vi "Test Enr file.vi"() -> ()   [LabVIEW 2021]
panel:
  out "Graphe XY 2":cluster{dbl[], dbl[]}(graph)
  in  "Booléen":bool
  out "Graphe XY":cluster{timestamp[], dbl[]}(graph)
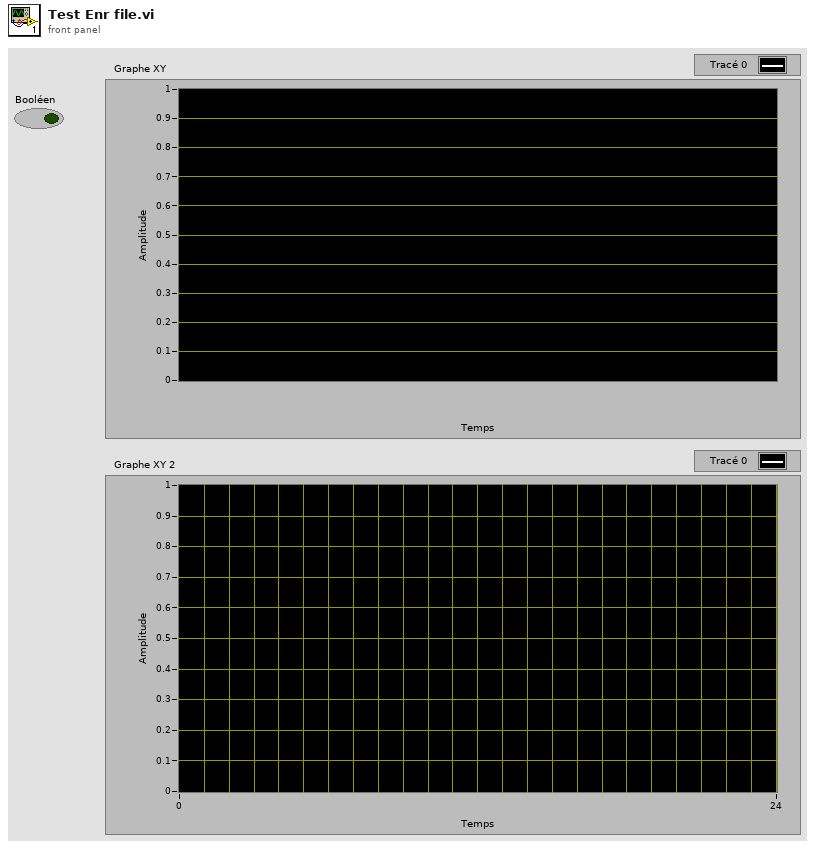
[diagram p1: front panel]
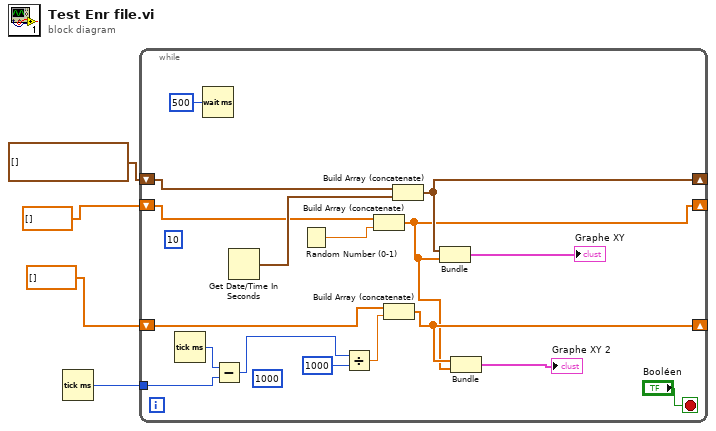
[diagram p0: block diagram]
diagram:
  n1 = Tick Count (ms)() -> (millisecond timer value=w1:u32)
  n2 = while {
    shift-right: [w17] -> _
    shift-left: timestamp[] [] -> [w19]
    shift-right: [w10] -> _
    shift-left: dbl[] [] -> [w16]
    shift-right: [w11] -> _
    shift-left: dbl[] [] -> [w14]
    tunnel: w1 -> [w12]
    stop <- "Booléen" stop-if-true
    (unwired) u32 1000 ("y")
    (unwired) 10
    n3 = Tick Count (ms)() -> (millisecond timer value=w13:u32)
    n4 = Wait (ms)(milliseconds to wait=u32 500 ("attente (ms)")) -> ()  [unwired: 1 out]
    n5 = Subtract(x=w13, y=w12) -> (x-y=w8:u32)
    n6 = Get Date/Time In Seconds() -> (seconds since 1Jan1904=w18:timestamp)
    n7 = Random Number (0-1)() -> (number: 0 to 1=w15:dbl)
    n8 = Divide(x=w8, y=u32 1000) -> (x/y=w6:dbl)
    n9 = Build Array (concatenate)(w16, w15) -> (w10:dbl[])
    n10 = Build Array (concatenate)(w14, w6) -> (w11:dbl[])
    n11 = Build Array (concatenate)(w19, w18) -> (w17:timestamp[])
    n12 = Bundle(w17, w10) -> (→"Graphe XY":cluster{timestamp[], dbl[]})  [unwired: 1 in]
    n13 = Bundle(w11, w10) -> (→"Graphe XY 2":cluster{dbl[], dbl[]})  [unwired: 1 in]
  }
